vi "act-0026-03-cor.vi"() -> ()   [LabVIEW 2010]
uses:
  lv_02/lv_02.lvlib
  lv_01/lv_01.lvlib
panel:
  out "F(tdeb)":dbl[](array[numeric])
  out "dN cum (t)":dbl[](array[numeric])
  in  "Effectif à t=0":u32
  out "f(tc)":dbl[](array[numeric])
  out "Graphe f(tc)":cluster{"tdeb":dbl[], "t":dbl[]}[](graph) caption="Graphe f(tc) et F(tdeb)"
  out "MTTF":dbl
  out "tc":dbl[](array[numeric])
  out "dN(tc)":u32[](array[numeric])
  out "tdeb":dbl[](array[numeric])
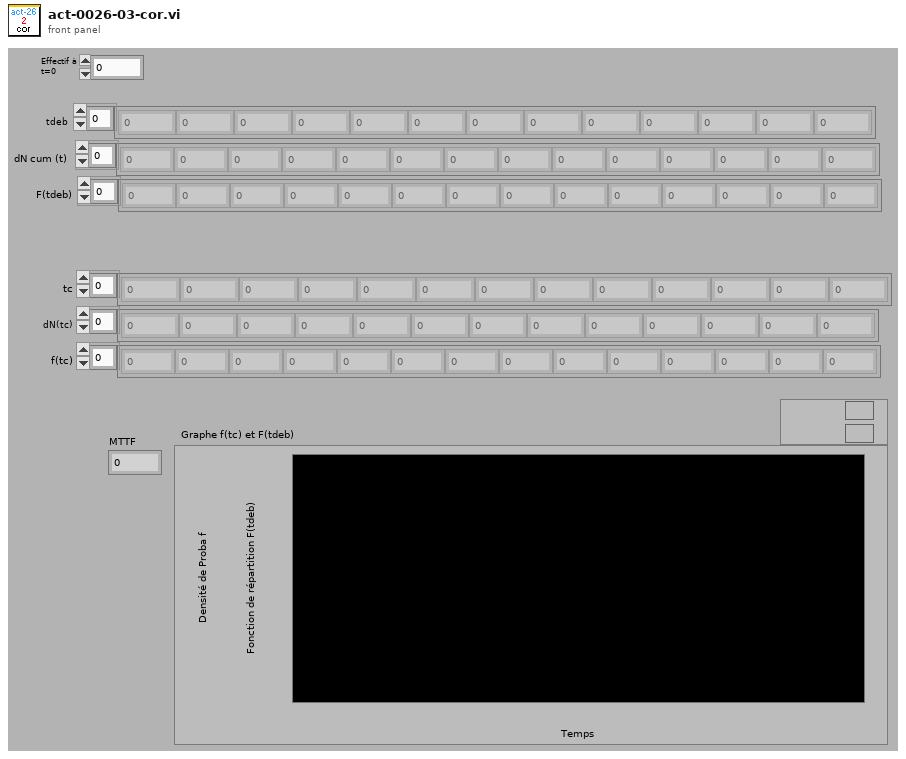
[diagram p1: front panel]
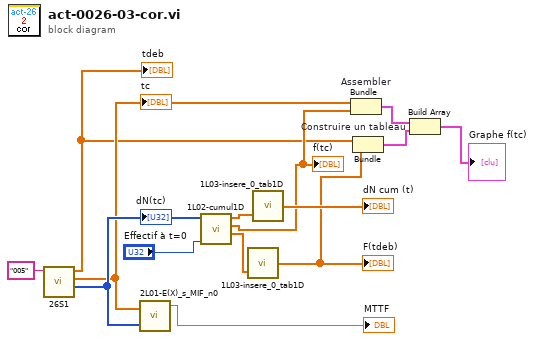
[diagram p0: block diagram]
diagram:
  n1 = call "26S1.vi"("src"="005") -> ("dN(tc)"=w12:u32[], "tc"=w8:dbl[], "tdeb"=w5:dbl[])  [unwired: 6 in, 2 out]
  "tdeb" <- w5
  "dN(tc)" <- w12
  "tc" <- w8
  n2 = call "2L01-E(X)_s_MIF_n0.vi"("ni"=w12, "xic"=w8) -> ("E(X)"=→"MTTF":dbl)  [unwired: 2 out]
  n3 = call "1L02-cumul1D.vi"("som_X"="Effectif à t=0", "X"=w12) -> ("X cum en %"=w1:dbl[], "X en %"=w7:dbl[], "X Cum"=w9:dbl[])  [unwired: 2 in, 1 out]
  "f(tc)" <- w7
  n4 = call "1L03-insere_0_tab1D.vi"("t"=w1) -> ("t"=w6:dbl[])  [unwired: 1 in]
  "F(tdeb)" <- w6
  n5 = call "1L03-insere_0_tab1D.vi"("t"=w9) -> ("t"=→"dN cum (t)":dbl[])  [unwired: 1 in]
  n6 = Bundle "Assembler"("tc"=w8, "X en %"=w7) -> (w4:cluster{"tc":dbl[], "X en %":dbl[]})  [unwired: 1 in]
  n7 = Bundle("tdeb"=w5, "t"=w6) -> (w3:cluster{"tdeb":dbl[], "t":dbl[]})  [unwired: 1 in]
  n8 = Build Array "Construire un tableau"(w4, w3) -> (→"Graphe f(tc)":cluster{"tdeb":dbl[], "t":dbl[]}[])
